vi "generate-analog-out-from-csv-file.vi"() -> ()   [LabVIEW 2020]
uses:
  <vilib>/Utility/error.llb/DialogType.ctl
  <vilib>/DAQmx/write.llb/DAQmx Write (Analog 1D DBL 1Chan NSamp).vi
  <vilib>/Utility/file.llb/Read From Spreadsheet File (DBL).vi
  <vilib>/DAQmx/create/channels.llb/DAQmx Create Channel (AO-Voltage-Basic).vi
  <vilib>/DAQmx/configure/timing.llb/DAQmx Timing (Use Waveform).vi
  <vilib>/DAQmx/miscellaneous.llb/DAQmx Fill In Error Info.vi
panel:
  in  "Column":i32
  in  "physical channels":tag="DAQ1/ao0"
  in  "error in":errorcluster
  out "error out":errorcluster
  in  "Delta T":dbl=0.0005
  in  "Sea State File":path=path "C:/data/analog-out-svm.csv"
  out "Waveform Graph":waveform(dbl)(graph) caption="Output Waveform"
  in  "Minimum Value":dbl format="%0.2f"
  in  "Maximum Value":dbl=5.0 format="%0.2f"
  in  "stop":bool
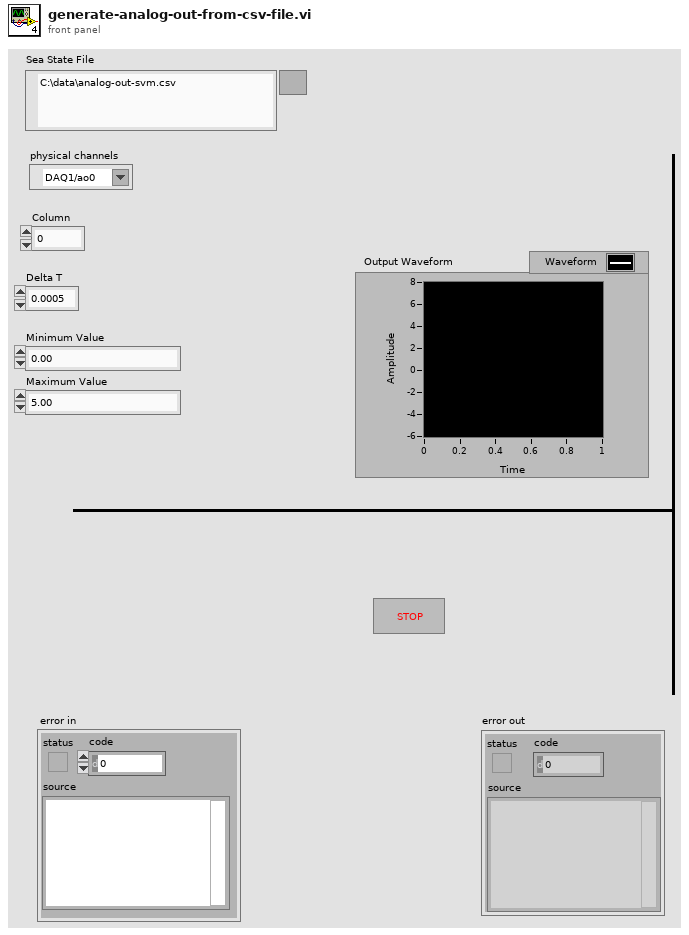
[diagram p1: front panel]
types:
  T1 = typedef "DialogType.ctl" = u16
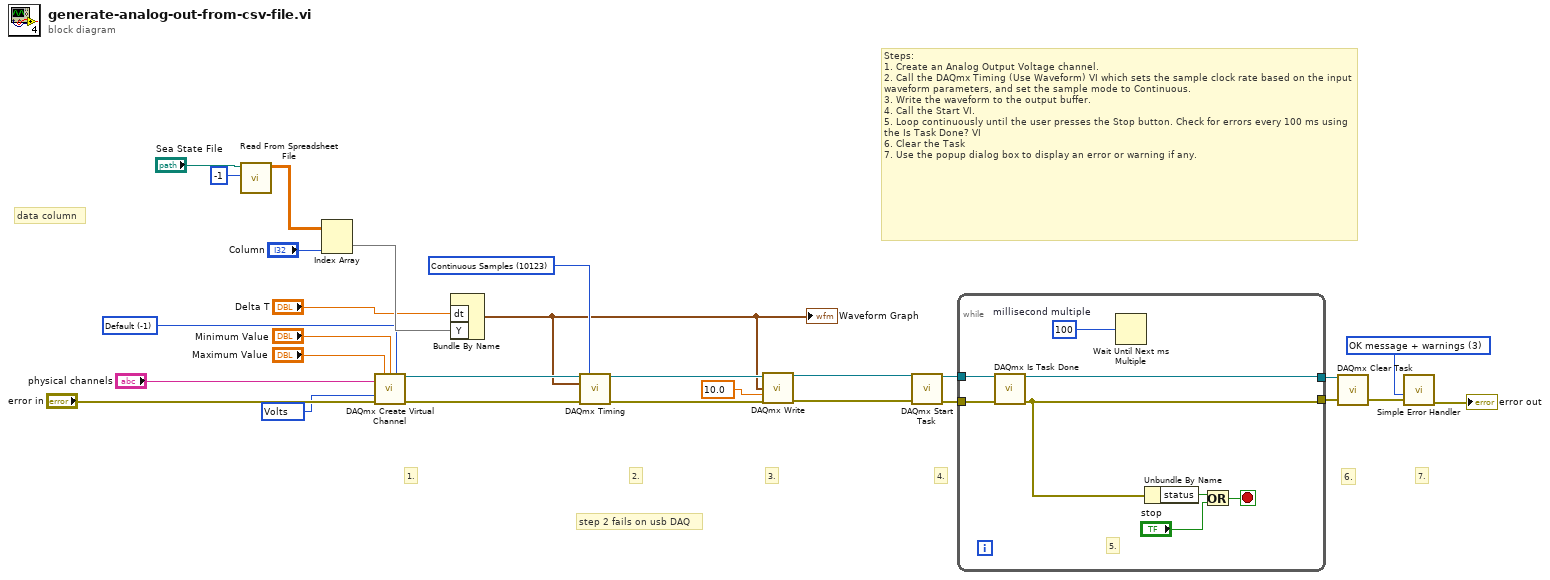
[diagram p0: block diagram]
diagram:
  w3 = 10348 items=["Volts"=10348, "From Custom Scale"=10065] ("units")
  w4 = -1 items=["Default"=-1, "RSE"=10083, "Differential"=10106, "Pseudodifferential"=12529] ("output terminal configuration")
  w17 = T1 3 items=["no dialog", "OK message", "continue or stop message", "OK message + warnings", "continue/stop + warnings"] ("type of dialog (OK msg:1)")
  w27 = 10123 items=["Finite Samples"=10178, "Continuous Samples"=10123] ("sample mode")
  # "data column"
  # "step 2 fails on usb DAQ"
  # "7."
  # "6."
  # "Steps: \n1. Create an Analog Output Voltage channel.\n2. Call the DAQmx Timing (Use Waveform) VI which sets the sample clock rate based on the input waveform parameters, and set the sample mode to Continuous.\n3. Write the waveform to the output buffer.\n4. Call the Start VI.\n5. Loop continuously until the user presses the Stop button. Check for errors every 100 ms using the Is Task Done? VI\n6. Clear the Task\n7. Use the popup dialog box to display an error or warning if any."
  # "4."
  # "3."
  # "2."
  # "1."
  n1 = call-poly <vilib>:"Read From Spreadsheet File.vi"("number of rows (all:-1)"=-1, "file path (dialog if empty)"="Sea State File") -> ("all rows"=w12:dbl[][])  [unwired: 5 in, 4 out]
  n2 = Index Array(array=w12, index (col)="Column") -> (element=w13:dbl[])  [unwired: 1 in]
  n3 = call-poly <vilib>:"DAQmx Create Virtual Channel.vi"("maximum value"="Maximum Value", "minimum value"="Minimum Value", "output terminal configuration"=w4, "physical channels"="physical channels", "units"=w3, "error in"="error in") -> ("task out"=w7:refnum<k21>, "error out"=w8:errorcluster)  [unwired: 8 in]
  n4 = Bundle By Name("dt"="Delta T", "Y"=w13) -> (w2:waveform(dbl))  [unwired: 1 in]
  "Waveform Graph" <- w2
  n5 = call-poly <vilib>:"DAQmx Timing.vi"("task/channels in"=w7, "sample mode"=w27, "waveform"=w2, "error in"=w8) -> ("task out"=w20:refnum<k21>, "error out"=w19:errorcluster)  [unwired: 10 in]
  n6 = call-poly <vilib>:"DAQmx Write.vi"("task/channels in"=w20, "data"=w2, "timeout"=10.0 ("Wirite Timeout"), "error in"=w19) -> ("task out"=w24:refnum<k21>, "error out"=w23:errorcluster)  [unwired: 9 in, 1 out]
  n7 = call <vilib>:"DAQmx Start Task.vi"("task/channels in"=w24, "error in"=w23) -> ("task out"=w18:refnum<k21>, "error out"=w21:errorcluster)  [unwired: 12 in]
  n8 = while {
    tunnel: w18 -> [w36]
    tunnel: [w35] -> w16
    tunnel: w21 -> [w34]
    tunnel: [w33] -> w15
    stop <- w31 stop-if-true
    w32 = u32 100  # millisecond multiple
    # "5."
    n9 = call <vilib>:"DAQmx Is Task Done.vi"("task/channels in"=w36, "error in"=w34) -> ("task out"=w35:refnum<k21>, "error out"=w33:errorcluster)  [unwired: 11 in, 1 out]
    n10 = Wait Until Next ms Multiple(millisecond multiple=w32) -> ()  [unwired: 1 out]
    n11 = Unbundle By Name(w33) -> ("status"=w30:bool)
    n12 = Or(x=w30, y="stop") -> (x .or. y?=w31:bool)
  }
  n13 = call <vilib>:"DAQmx Clear Task.vi"("task in"=w16, "error in"=w15) -> ("error out"=w28:errorcluster)  [unwired: 13 in]
  n14 = call <vilib>:"Simple Error Handler.vi"("type of dialog (OK msg:1)"=w17, "error in (no error)"=w28) -> ("error out"=→"error out":errorcluster)  [unwired: 3 in, 4 out]
